vi "VG-init.vi"(8 "error in (no error)":errorcluster, 11 "VG-VNA_GUI in":refnum<class "VG-VNA_GUI.lvclass">) -> (0 "error out":errorcluster, 3 "VG-VNA_GUI out":refnum<class "VG-VNA_GUI.lvclass">)   [LabVIEW 2020, in "VG-VNA_GUI.lvlib" / "VG-VNA_GUI.lvclass"]
uses:
  VG-VNA_GUI.lvclass
  C:/Program Files (x86)/National Instruments/LabVIEW 2020/vi.lib/ActorFramework/Actor/Actor.lvclass
  data_handler/VDH-VNA_data_handler/VDH-VNA_data_handler/VDH-preLaunchConfig.ctl
  data_handler/VDH-VNA_data_handler/VDH-VNA_data_handler/VDH-actor_enqueues.ctl
  <vilib>/ActorFramework/Message Enqueuer/Message Enqueuer.lvclass
  hardware_manager/VHM-VNA_Hardware_Manager/VHM-VNA_Hardware_Manager/VHM-preLaunchConfig.ctl
  <vilib>/ActorFramework/Actor/Actor.lvclass/Actor.ctl
  <vilib>/ActorFramework/Message Enqueuer/Message Enqueuer.lvclass/Message Enqueuer.ctl
  VG-VNA_GUI.lvclass/VG-VNA_GUI.ctl
  <vilib>/ActorFramework/Message Enqueuer/Init from Existing Queue.vi
  hardware_manager/VHM-VNA_Hardware_Manager/VHM-VNA_Hardware_Manager/VHM-VNA_Hardware_Manager.lvclass
  data_handler/VDH-VNA_data_handler/VDH-VNA_data_handler/VDH-VNA_data_handler.lvclass
  <vilib>/ActorFramework/Actor/Actor.lvclass
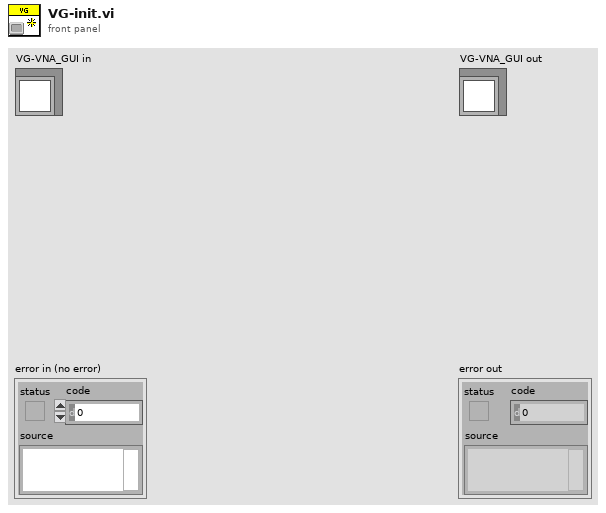
[diagram p1: front panel]
types:
  T1 = typedef "VHM-VNA_Hardware_Manager.lvlib/VHM-VNA_Hardware_Manager.lvclass/VHM-preLaunchConfig.ctl" = cluster{"UI":refnum<class "Message Enqueuer.lvclass">}
  T2 = typedef "VDH-VNA_data_handler.lvlib/VDH-VNA_data_handler.lvclass/VDH-preLaunchConfig.ctl" = cluster{"AF enq":T3}
  T3 = typedef "VDH-VNA_data_handler.lvlib/VDH-VNA_data_handler.lvclass/VDH-actor_enqueues.ctl" = cluster{"UI":refnum<class "Message Enqueuer.lvclass">, "HWM":refnum<class "Message Enqueuer.lvclass">}
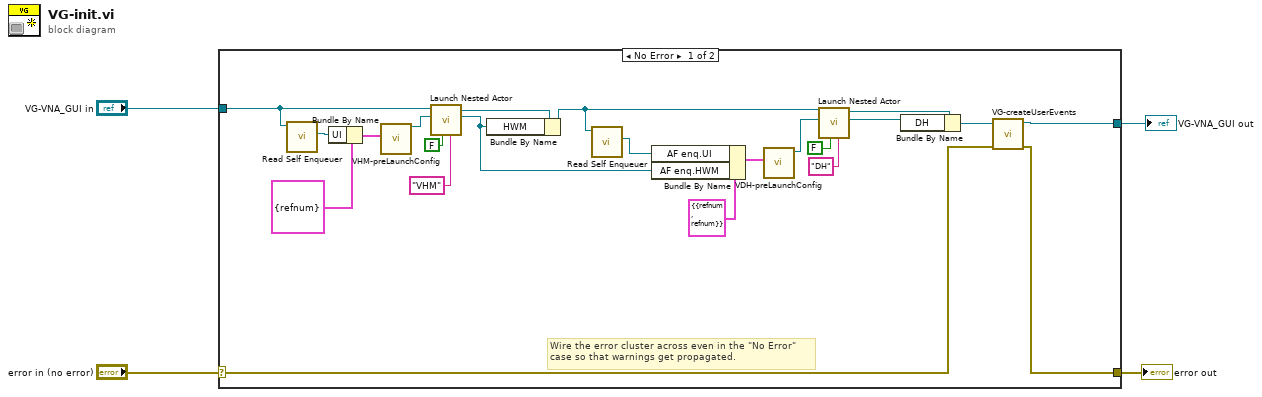
[diagram p0: block diagram]
diagram:
  n1 = case shown="No Error" "error in (no error)" {
    selector: "error in (no error)" -> [w10 w28]
    tunnel: [w9 w28] -> w3
    tunnel: [w11 w27] -> w1
    tunnel: "VG-VNA_GUI in" -> [w16 w27]
    frame No Error {
      # "Wire the error cluster across even in the \"No Error\"\ncase so that warnings get propagated."
      n2 = call <vilib>:"Read Self Enqueuer.vi"("Actor"=w16) -> ("Self Enqueuer"=w15:refnum<class "Message Enqueuer.lvclass">)  [unwired: 10 in]
      n3 = Bundle By Name(cluster=T1 {"UI"=refnum} ("preLaunchConfig"), "UI"=w15) -> (w17:T1)
      n4 = call "VHM-preLaunchConfig.vi"("preLaunchConfig"=w17) -> ("VHM-VNA_Hardware_Manager out"=w22:refnum<class "VHM-VNA_Hardware_Manager.lvclass">)  [unwired: 10 in]
      n5 = call <vilib>:"Launch Nested Actor.vi"("Debug Alias"="VHM", "Open Actor Core front panel? (F)"=FALSE, "Nested Actor"=w22, "Caller Actor in"=w16) -> ("Nested Actor's Enqueuer"=w20:refnum<class "Message Enqueuer.lvclass">, "Caller Actor out"=w26:refnum<class "VG-VNA_GUI.lvclass">)  [unwired: 5 in, 1 out]
      n6 = Bundle By Name(cluster=w26, "HWM"=w20) -> (w19:refnum<class "VG-VNA_GUI.lvclass">)
      n7 = call <vilib>:"Read Self Enqueuer.vi"("Actor"=w19) -> ("Self Enqueuer"=w18:refnum<class "Message Enqueuer.lvclass">)  [unwired: 10 in]
      n8 = Bundle By Name(cluster=T2 {"AF enq"={"UI"=refnum, "HWM"=refnum}} ("preLauch Config"), "AF enq.UI"=w18, "AF enq.HWM"=w20) -> (w23:T2)
      n9 = call "VDH-preLaunchConfig.vi"("preLauch Config"=w23) -> ("VDH-VNA_data_handler out"=w25:refnum<class "VDH-VNA_data_handler.lvclass">)  [unwired: 10 in]
      n10 = call <vilib>:"Launch Nested Actor.vi"("Debug Alias"="DH", "Open Actor Core front panel? (F)"=FALSE, "Nested Actor"=w25, "Caller Actor in"=w19) -> ("Nested Actor's Enqueuer"=w13:refnum<class "Message Enqueuer.lvclass">, "Caller Actor out"=w14:refnum<class "VG-VNA_GUI.lvclass">)  [unwired: 5 in, 1 out]
      n11 = Bundle By Name(cluster=w14, "DH"=w13) -> (w12:refnum<class "VG-VNA_GUI.lvclass">)
      n12 = call "VG-createUserEvents.vi"("error in (no error)"=w10, "VG-VNA_GUI in"=w12) -> ("error out"=w9:errorcluster, "VG-VNA_GUI out"=w11:refnum<class "VG-VNA_GUI.lvclass">)  [unwired: 8 in]
    }
    frame Error {
    }
  }
  "error out" <- w3
  "VG-VNA_GUI out" <- w1
